vi "Simulation Driver.vi"() -> ()   [LabVIEW 2019]
uses:
  subVIs/Global Variables.vi
panel:
  in  "Data Queue":refnum<queue>
  in  "Background Image":refnum<vi>
  in  "Inkscape File (.svg)":refnum<vi>
  in  "Run":refnum<vi>
  in  "Abort":refnum<vi>
  in  "Lithography Data":T1(array[cluster])
  # "Usually these controls will be hidden\nand settings will be displayed here."
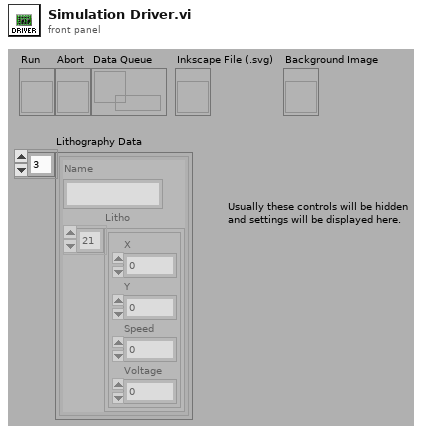
[diagram p1: front panel]
types:
  T1 = cluster{"Name":string, "Litho":cluster{"X":dbl, "Y":dbl, "Speed":dbl, "Voltage":dbl}[]}[]
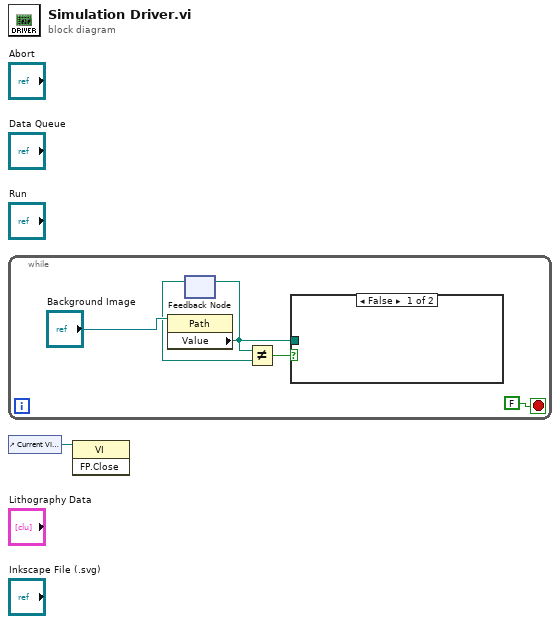
[diagram p0: block diagram]
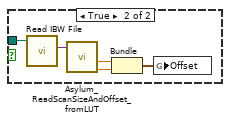
[diagram p2: hidden frame]
diagram:
  n1 = while {
    stop <- FALSE stop-if-true
    n2 = property class="Path"(reference="Background Image") -> ("Value"=w4:path)  [unwired: 1 in, 2 out]
    n3 = feedback #1() -> (w2:path)  [unwired: 1 in]
    n4 = feedback-in #1(w4) -> ()
    n5 = Not Equal?(x=w4, y=w2) -> (x != y?=w3:bool)
    n6 = case shown="False" w3 {
      tunnel: w4 -> [_ w9]
      frame False {
      }
      frame True {
        n7 = call "Read IBW File.vi"("Path"=w9) -> ("Notes LUT"=w10:variant)  [unwired: 8 in, 2 out]
        n8 = call "Asylum_ReadScanSizeAndOffset_fromLUT.vi"("Notes LUT"=w10) -> ("Y Offset"=w7:dbl, "X Offset"=w8:dbl)  [unwired: 7 in, 2 out]
        n9 = Bundle("X Offset"=w8, "Y Offset"=w7) -> (w11:cluster{"X Offset":dbl, "Y Offset":dbl})  [unwired: 1 in]
        n10 = global write "Global Variables.vi" "Offset"(w11) -> ()
      }
    }
  }
  n11 = control-ref of="Current VI Reference"() -> (w1:refnum<vi>)
  n12 = invoke class="VI" method="FP.Close"(reference=w1) -> ()  [unwired: 2 in, 3 out]
